vi "Handler - StartStop Acquisition.vi"(8 "error in (no error)":errorcluster, 10 "Input Acquisition Period":i64, 11 "Message Handler Loop Data in":T1) -> (0 "error out":errorcluster, 2 "Acquisition Period out":i64, 3 "Message Handler Loop Data out":T1)   [LabVIEW 2018]
uses:
  RT - Instrument IO.lvlib
  Variables/Global - cRIO Configuration Options.vi
  <vilib>/gmath/NI_Gmath.lvlib
  Private Controls/Message Handler Loop Data.ctl
  FPGA/FPGA VI Reference.ctl
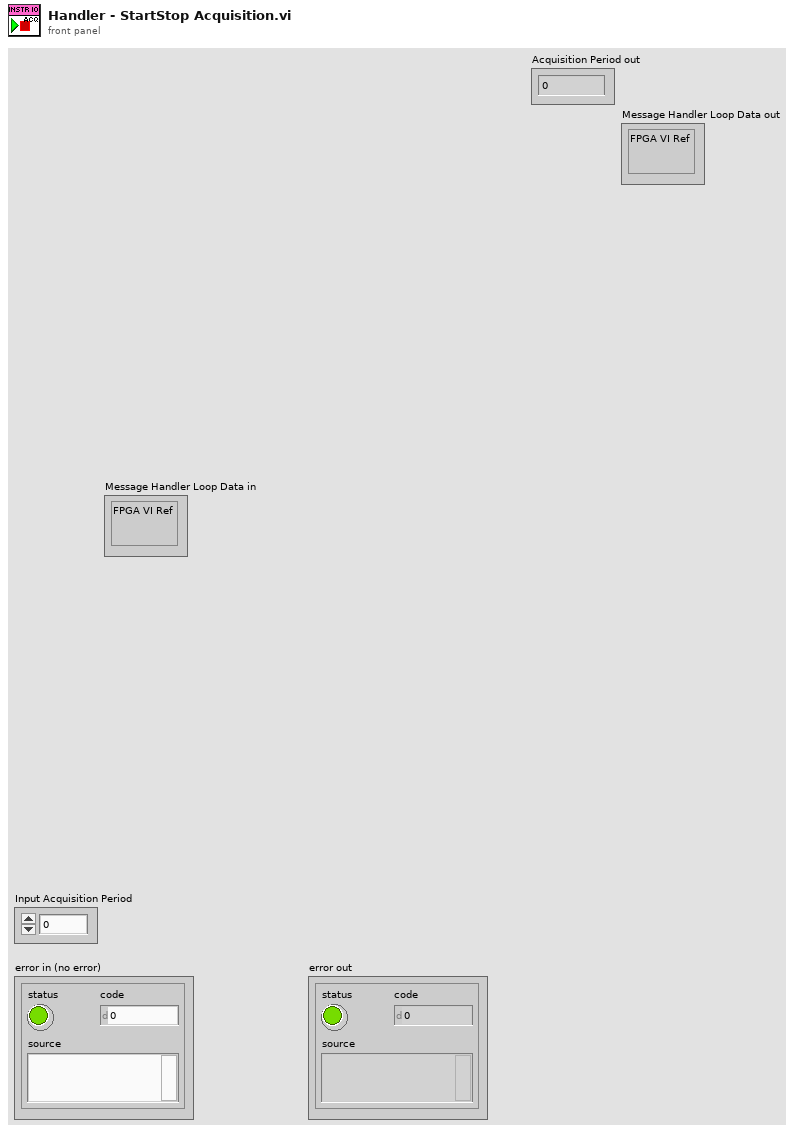
[diagram p1: front panel]
types:
  T1 = typedef "RT - Instrument IO.lvlib/Message Handler Loop Data.ctl" = cluster{"FPGA VI Ref":T2}
  T2 = typedef "FPGA VI Reference.ctl" = refnum<k20>
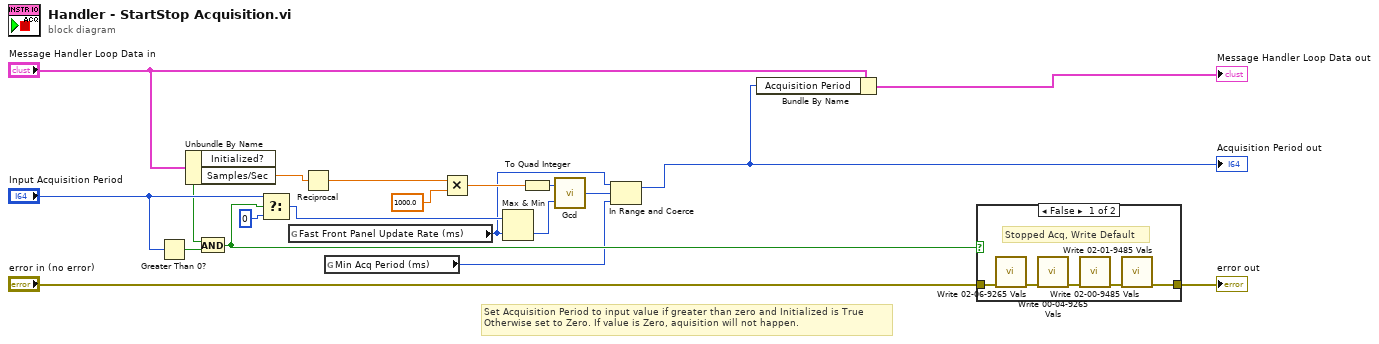
[diagram p0: block diagram]
diagram:
  # "Set Acquisition Period to input value if greater than zero and Initialized is True\nOtherwise set to Zero. If value is Zero, aquisition will not happen."
  n1 = Greater Than 0?(x="Input Acquisition Period") -> (x > 0?=w16:bool)
  n2 = Unbundle By Name("Message Handler Loop Data in") -> ("Initialized?"=w15:bool, "Samples/Sec"=w9:dbl)
  n3 = And(x=w15, y=w16) -> (x .and. y?=w8:bool)
  n4 = Select(t="Input Acquisition Period", s=w8, f=i64 0) -> (s? t:f=w7:i64)
  n5 = global read "Global - cRIO Configuration Options.vi" "Fast Front Panel Update Rate (ms)"() -> (w2:i32)
  n6 = Reciprocal(x=w9) -> (1/x=w12:dbl)
  n7 = global read "Global - cRIO Configuration Options.vi" "Min Acq Period (ms)"() -> (w1:i32)
  n8 = Multiply(x=w12, y=1000.0) -> (x*y=w10:dbl)
  n9 = Max & Min(x=w7, y=w2) -> (min(x,y)=w5:i64)  [unwired: 1 out]
  n10 = To Quad Integer(1:w10) -> (0:w6:i64)
  n11 = call <vilib>:"Gcd.vi"("y"=w5, "x"=w6) -> ("gcd(x,y)"=w4:i32)
  n12 = In Range and Coerce(upper limit=w2, x=w4, lower limit=w1) -> (coerced(x)=w3:i32)  [unwired: 1 out]
  "Acquisition Period out" <- w3
  n13 = Bundle By Name(cluster="Message Handler Loop Data in", "Acquisition Period"=w3) -> (→"Message Handler Loop Data out":T1)
  n14 = case shown="False" w8 {
    tunnel: "error in (no error)" -> [w21 w26]
    tunnel: [w22 w26] -> w20
    frame False {
      # "Stopped Acq, Write Default"
      n15 = call "Write 02-06-9265 Vals.vi"("error in (no error)"=w21) -> ("error out"=w23:errorcluster)  [unwired: 10 in]
      n16 = call "Write 00-04-9265 Vals.vi"("error in (no error)"=w23) -> ("error out"=w24:errorcluster)  [unwired: 10 in]
      n17 = call "Write 02-00-9485 Vals.vi"("error in (no error)"=w24) -> ("error out"=w25:errorcluster)  [unwired: 10 in]
      n18 = call "Write 02-01-9485 Vals.vi"("error in (no error)"=w25) -> ("error out"=w22:errorcluster)  [unwired: 10 in]
    }
    frame True {
      # "Started Acq"
    }
  }
  "error out" <- w20
